vi "lowpass1.vi"(8 "Error In":errorcluster, 9 "SignalInput":refnum<class "DoublePointer.lvclass">, 10 "elementsCount":i16, 11 "SigalOutput":refnum<class "DoublePointer.lvclass">) -> (0 "Error Out":errorcluster)   [LabVIEW 2014]
uses:
  <vilib>/LabVIEW Universal Transcriptor/LabVIEW to Arduino Transcriptor/Transcriptors/System API/Basic Datatypes Pointers/DoublePointer.lvclass
  <vilib>/measure/NI_MABase.lvlib
  utils/DLL InputOutput/DLL InputOutput Lib.lvlib
panel:
  out "DEBUG samples out":string
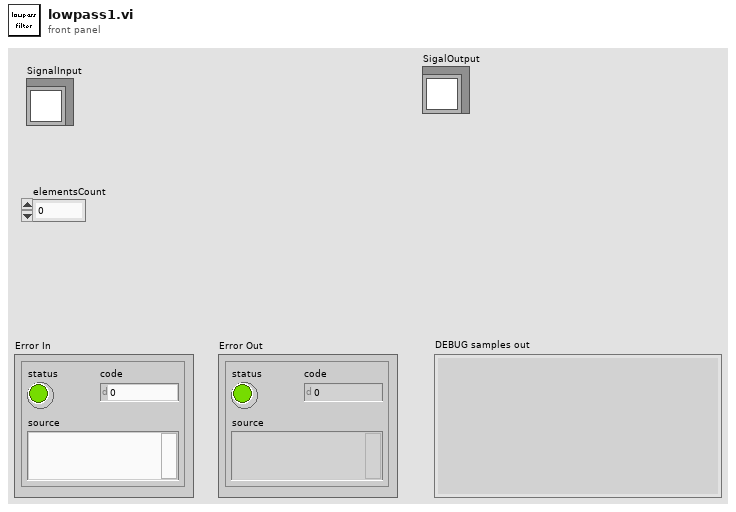
[diagram p1: front panel]
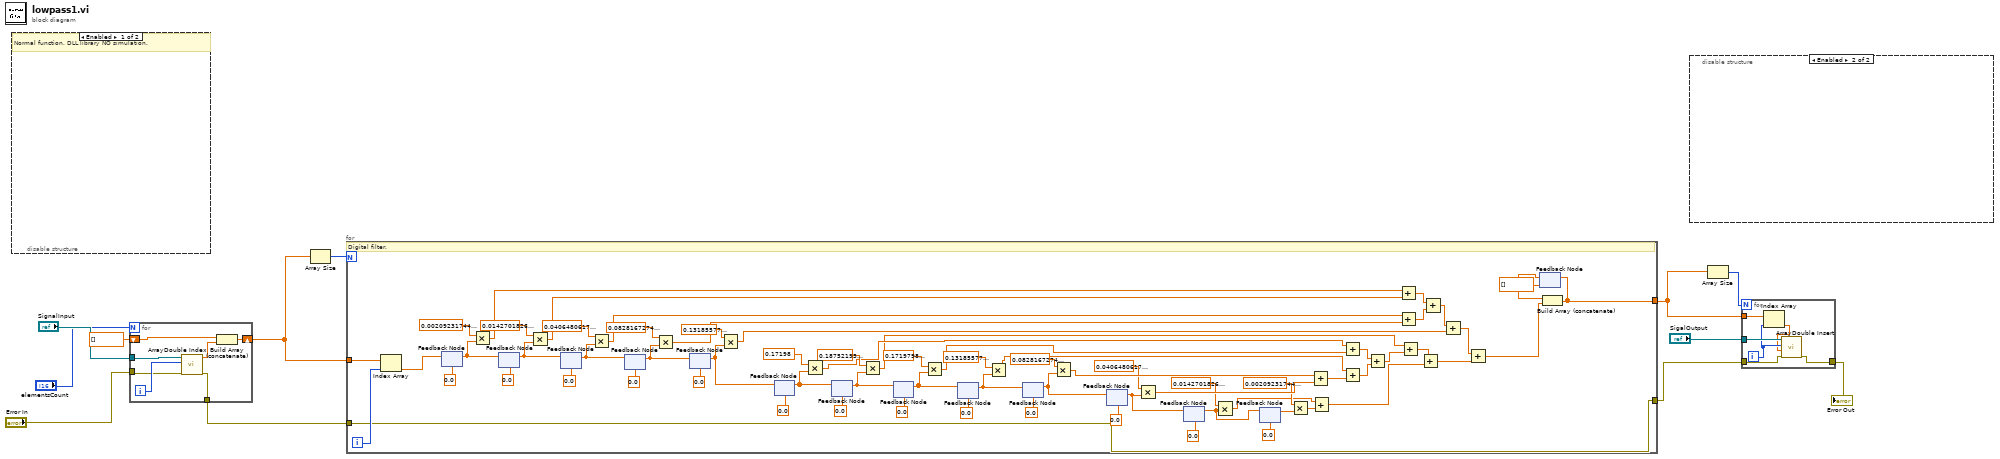
[diagram p0: block diagram]
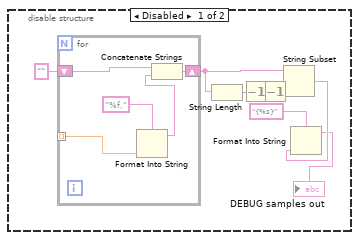
[diagram p2: hidden frame]
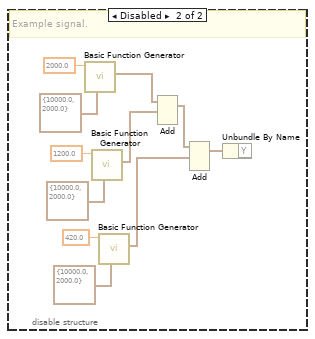
[diagram p3: hidden frame]
diagram:
  n1 = disable-structure "Diagram Disable Structure" shown="Enabled" {
    frame Enabled {
      # "Normal function, DLL library NO simulation."
    }
    frame Disabled {
      # "Example signal."
      n2 = call <vilib>:"Basic Function Generator.vi"("sampling info"=cluster{"Fs":dbl, "#s":dbl} {"Fs"=10000.0, "#s"=2000.0}, "frequency"=2000.0) -> ("signal out"=w17:waveform(dbl))  [unwired: 7 in, 2 out]
      n3 = call <vilib>:"Basic Function Generator.vi"("sampling info"=cluster{"Fs":dbl, "#s":dbl} {"Fs"=10000.0, "#s"=2000.0}, "frequency"=1200.0) -> ("signal out"=w16:waveform(dbl))  [unwired: 7 in, 2 out]
      n4 = call <vilib>:"Basic Function Generator.vi"("sampling info"=cluster{"Fs":dbl, "#s":dbl} {"Fs"=10000.0, "#s"=2000.0}, "frequency"=420.0) -> ("signal out"=w15:waveform(dbl))  [unwired: 7 in, 2 out]
      n5 = Add(1:w16, 2:w17) -> (0:w18:waveform(dbl))  [unwired: 1 in, 1 out]
      n6 = Add(1:w15, 2:w18) -> (0:w14:waveform(dbl))  [unwired: 1 in, 1 out]
      n7 = Unbundle By Name(w14) -> ("Y"=w13:dbl[])
    }
  }
  n8 = for {
    N: "elementsCount" -> [_]
    tunnel: "SignalInput" -> [w31]
    tunnel: "Error In" -> [w29]
    shift-right: [w27] -> w6
    shift-left: dbl[] [] -> [w26]
    tunnel: [w25] -> w7
    i -> [w30]
    n9 = call "ArrayDouble Index.vi"("Error In"=w29, "index"=w30, "DoublePointer.lvclass"=w31) -> ("Error Out"=w25:errorcluster, "element"=w28:dbl)  [unwired: 7 in]
    n10 = Build Array (concatenate)(w26, w28) -> (w27:dbl[])
  }
  n11 = Array Size(array=w6) -> (size(s)=w12:i32)
  n12 = for {
    N: w12 -> [_]
    tunnel: w6 -> [w102]
    tunnel: [w77] -> w1
    tunnel: w7 -> [w33]
    tunnel: [w33] -> w5
    i -> [w101]
    # "Digital filter."
    n13 = Index Array(array=w102, index=w101) -> (element=w100:dbl)
    n14 = feedback-in #1(w100) -> ()
    n15 = feedback #1(0.0 ("number out")) -> (w91:dbl)
    n16 = Multiply(x=0.002092317445203662, y=w91) -> (x*y=w86:dbl)
    n17 = feedback #2(0.0 ("number out")) -> (w90:dbl)
    n18 = feedback-in #2(w91) -> ()
    n19 = Multiply(x=0.014270182698965073, y=w90) -> (x*y=w85:dbl)
    n20 = feedback #3(0.0 ("number out")) -> (w89:dbl)
    n21 = feedback-in #3(w90) -> ()
    n22 = Multiply(x=0.04064806178212166, y=w89) -> (x*y=w84:dbl)
    n23 = feedback #4(0.0 ("number out")) -> (w82:dbl)
    n24 = feedback-in #4(w89) -> ()
    n25 = Multiply(x=0.0828167274594307, y=w82) -> (x*y=w81:dbl)
    n26 = feedback #5(0.0 ("number out")) -> (w62:dbl)
    n27 = feedback-in #5(w82) -> ()
    n28 = Multiply(x=0.131855770945549, y=w62) -> (x*y=w79:dbl)
    n29 = feedback #6(0.0 ("number out")) -> (w68:dbl)
    n30 = feedback-in #6(w62) -> ()
    n31 = Multiply(x=0.17198, y=w68) -> (x*y=w58:dbl)
    n32 = feedback #7(0.0 ("number out")) -> (w67:dbl)
    n33 = feedback-in #7(w68) -> ()
    n34 = Multiply(x=0.18752193450927734, y=w67) -> (x*y=w54:dbl)
    n35 = feedback #8(0.0 ("number out")) -> (w66:dbl)
    n36 = feedback-in #8(w67) -> ()
    n37 = Multiply(x=0.1719798743724823, y=w66) -> (x*y=w57:dbl)
    n38 = feedback #9(0.0 ("number out")) -> (w64:dbl)
    n39 = feedback-in #9(w66) -> ()
    n40 = Multiply(x=0.131855770945549, y=w64) -> (x*y=w56:dbl)
    n41 = feedback #10(0.0 ("number out")) -> (w48:dbl)
    n42 = feedback-in #10(w64) -> ()
    n43 = Multiply(x=0.0828167274594307, y=w48) -> (x*y=w52:dbl)
    n44 = feedback #11(0.0 ("number out")) -> (w40:dbl)
    n45 = feedback-in #11(w48) -> ()
    n46 = Multiply(x=0.04064806178212166, y=w40) -> (x*y=w49:dbl)
    n47 = feedback #12(0.0 ("number out")) -> (w39:dbl)
    n48 = feedback-in #12(w40) -> ()
    n49 = Multiply(x=0.014270182698965073, y=w39) -> (x*y=w42:dbl)
    n50 = feedback #13(0.0 ("number out")) -> (w43:dbl)
    n51 = feedback-in #13(w39) -> ()
    n52 = Multiply(x=0.002092317445203662, y=w43) -> (x*y=w41:dbl)
    n53 = Add(x=w52, y=w49) -> (x+y=w53:dbl)
    n54 = Add(x=w42, y=w41) -> (x+y=w36:dbl)
    n55 = Add(x=w58, y=w57) -> (x+y=w61:dbl)
    n56 = Add(x=w56, y=w53) -> (x+y=w60:dbl)
    n57 = Add(x=w61, y=w60) -> (x+y=w55:dbl)
    n58 = Add(x=w86, y=w85) -> (x+y=w87:dbl)
    n59 = Add(x=w84, y=w81) -> (x+y=w88:dbl)
    n60 = Add(x=w54, y=w55) -> (x+y=w38:dbl)
    n61 = Add(x=w38, y=w36) -> (x+y=w37:dbl)
    n62 = Add(x=w87, y=w88) -> (x+y=w80:dbl)
    n63 = Add(x=w80, y=w79) -> (x+y=w59:dbl)
    n64 = Add(x=w59, y=w37) -> (x+y=w32:dbl)
    n65 = feedback #14(dbl[] []) -> (w34:dbl[])
    n66 = Build Array (concatenate)(w34, w32) -> (w77:dbl[])
    n67 = feedback-in #14(w77) -> ()
  }
  n68 = disable-structure "Diagram Disable Structure" shown="Enabled" {
    frame Disabled {
      n69 = for {
        tunnel: [w115] -> w111 mode=indexing
        shift-right: [w113] -> w109
        shift-left: "" -> [w112]
        n70 = Format Into String(format string="%f,", w115) -> (resulting string=w114:string)  [unwired: 2 in, 1 out]
        n71 = Concatenate Strings(w112, w114) -> (w113:string)
      }
      n72 = String Length(string=w109) -> (length=w108:i32)
      n73 = Decrement(x=w108) -> (x-1=w106:i32)
      n74 = Decrement(x=w106) -> (x-1=w107:i32)
      n75 = String Subset(string=w109, length (rest)=w107) -> (substring=w104:string)  [unwired: 1 in]
      n76 = Format Into String(format string="{%s}", w104) -> (resulting string=→"DEBUG samples out":string)  [unwired: 2 in, 1 out]
    }
    frame Enabled {
    }
  }
  n77 = Array Size(array=w1) -> (size(s)=w2:i32)
  n78 = for {
    N: w2 -> [_]
    tunnel: "SigalOutput" -> [w120]
    tunnel: w5 -> [w122]
    tunnel: [w121] -> w4
    tunnel: w1 -> [w119]
    i -> [w118]
    n79 = Index Array(array=w119, index=w118) -> (element=w117:dbl)
    n80 = call "ArrayDouble Insert.vi"("Error In"=w122, "element"=w117, "index"=w118, "DoublePointer.lvclass"=w120) -> ("Error Out"=w121:errorcluster)  [unwired: 7 in]
  }
  "Error Out" <- w4
